vi "Stop Core.vi"(10 "final error code":i32, 11 "Jobber Proxy in":refnum<class "Jobber Proxy.lvclass">) -> (3 "Jobber Proxy out":refnum<class "Jobber Proxy.lvclass">)   [LabVIEW 2014, in "Jobber Proxy.lvlib" / "Jobber Proxy.lvclass"]
doc: "(<B>Filename</B>: Actor Framework.lvlib:Actor.lvclass:Stop Core.vi)\n\nDefines what the actor does before it stops. Use the <B>final error code</B> input to determine whether the actor shut down in response to an error.\n\nBy default, this method does nothing. A descendant class may override it to define behavior, such as shutting down any processes the actor initiated in its override of the Actor Core method."
uses:
  Jobber Proxy.lvclass
  Jobber Proxy.lvclass/Jobber Proxy.ctl
  <vilib>/ActorFramework/Stop Msg/Stop Msg.lvclass/Stop Msg.ctl
  <vilib>/ActorFramework/Message Enqueuer/Message Enqueuer.lvclass/Message Enqueuer.ctl
  <vilib>/ActorFramework/Stop Msg/Send Emergency Stop.vi
  <vilib>/ActorFramework/Stop Msg/Send Normal Stop.vi
  <vilib>/ActorFramework/Message Enqueuer/Enqueue Critical.vi
  <vilib>/ActorFramework/Message Enqueuer/Enqueue.vi
  <vilib>/ActorFramework/Message Priority Queue/Priority Enqueue.vi
  <vilib>/ActorFramework/Actor/Actor.lvclass
  <vilib>/ActorFramework/Stop Msg/Stop Msg.lvclass
  Classes/LabVIEW Instance/LabVIEW Instance.lvclass
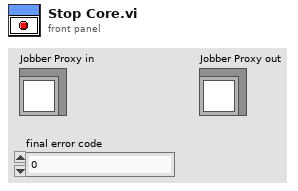
[diagram p1: front panel]
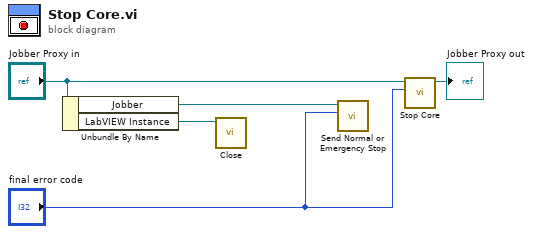
[diagram p0: block diagram]
diagram:
  n1 = Unbundle By Name("Jobber Proxy in") -> ("Jobber"=w3:refnum<class "Message Enqueuer.lvclass">, "LabVIEW Instance"=w1:refnum<class "LabVIEW Instance.lvclass">)
  n2 = call "Close.vi"("LabVEIW Instance in"=w1) -> ()  [unwired: 10 in, 1 out]
  n3 = call <vilib>:"Send Normal or Emergency Stop.vi"("final error code"="final error code", "Message Enqueuer"=w3) -> ()  [unwired: 9 in, 1 out]
  n4 = call-parent "Stop Core.vi"("final error code"="final error code", "Actor in"="Jobber Proxy in") -> ("Actor out"=→"Jobber Proxy out":refnum<class "Jobber Proxy.lvclass">)  [unwired: 9 in]
